vi "AutoAdjustCamera.vi"(8 "error in":errorcluster, 10 "Camera Settings":T1={"Brightness"=150, "Contrast"=0.2, "Threshold"=0.2}, 11 "Session In":T2) -> (0 "error out":errorcluster, 1 "Brightness":i64, 2 "Contrast":dbl, 3 "Session Out":T2, 4 "All Edges Found":bool, 5 "Threshold":sgl)   [LabVIEW 2017]
uses:
  <vilib>/userdefined/High Color/IMAQdx.ctl
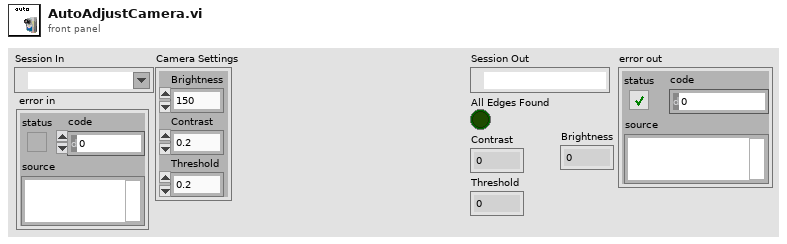
[diagram p1: front panel]
types:
  T1 = cluster{"Brightness":i64, "Contrast":dbl, "Threshold":sgl}
  T2 = typedef "IMAQdx.ctl" = refnum<k21>
  T3 = typedef "IMAQ Coordinate System" = cluster{"Reference System":cluster{"Origin":cluster{"X":sgl, "Y":sgl}, "Angle (deg)":sgl, "Axis Reference":u32}, "Measurement System":cluster{"Origin":cluster{"X":sgl, "Y":sgl}, "Angle (deg)":sgl, "Axis Reference":u32}}
  T4 = typedef "IMAQ Image.ctl" = refnum<image>
  T5 = cluster{"Point1 (Pixels)":cluster{"X":sgl, "Y":sgl}, "Point2 (Pixels)":cluster{"X":sgl, "Y":sgl}, "Point1 (Real-World)":cluster{"X":sgl, "Y":sgl}, "Point2 (Real-World)":cluster{"X":sgl, "Y":sgl}, "Angle (Pixel)":dbl, "Angle (Real-World)":dbl, "Score":dbl, "Straightness":dbl, "Average SNR (db)":dbl, "Calibration Valid":bool}[]
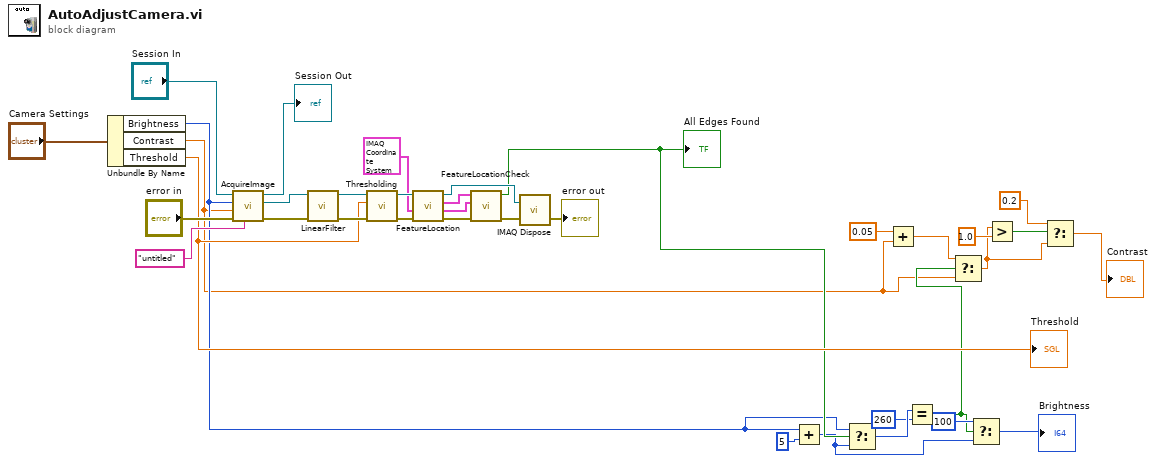
[diagram p0: block diagram]
diagram:
  n1 = Unbundle By Name("Camera Settings") -> ("Brightness"=w15:i64, "Contrast"=w8:dbl, "Threshold"=w20:sgl)
  "Threshold" <- w20
  n2 = call "AcquireImage.vi"("Image Name"="untitled", "error in"="error in", "Contrast"=w8, "Brightness"=w15, "Session In"="Session In") -> ("error out"=w32:errorcluster, "Image"=w31:T4, "Session Out"=→"Session Out":T2)  [unwired: 3 in]
  n3 = call "LinearFilter.vi"("error in (no error)"=w32, "Image Src"=w31) -> ("error out"=w26:errorcluster, "Image"=w25:T4)  [unwired: 8 in]
  n4 = call "Thresholding.vi"("error in (no error)"=w26, "Threshold Value"=w20, "Image Src"=w25) -> ("error out"=w28:errorcluster, "Image"=w27:T4)  [unwired: 7 in]
  n5 = call "FeatureLocation.vi"("error in (no error)"=w28, "Coordinate System"=T3 {"Reference System"={"Origin"={"X"=0.0, "Y"=0.0}, "Angle (deg)"=0.0, "Axis Reference"=0}, "Measurement System"={"Origin"={"X"=0.0, "Y"=0.0}, "Angle (deg)"=0.0, "Axis Reference"=0}}, "Image"=w27) -> ("error out"=w33:errorcluster, "Vertical Edges"=w30:T5, "Horizontal Edges"=w29:T5, "Image 2"=w35:T4)  [unwired: 3 in, 2 out]
  n6 = call "FeatureLocationCheck.vi"("error in (no error)"=w33, "Vertical Edges"=w30, "Horizontal Edges"=w29) -> ("error out"=w34:errorcluster, "All Edges Found"=w16:bool)  [unwired: 7 in]
  "All Edges Found" <- w16
  n7 = call "IMAQ Dispose"("Image"=w35, "error in (no error)"=w34) -> ("error out"=→"error out":errorcluster)  [unwired: 4 in]
  n8 = Add(x=w15, y=i64 5) -> (x+y=w11:i64)
  n9 = Select(t=w15, s=w16, f=w11) -> (s? t:f=w14:i64)
  n10 = Add(x=0.05, y=w8) -> (x+y=w6:dbl)
  n11 = Equal?(x=w14, y=i64 260) -> (x = y?=w9:bool)
  n12 = Select(t=w6, s=w9, f=w8) -> (s? t:f=w2:dbl)
  n13 = Select(t=i64 100, s=w9, f=w11) -> (s? t:f=→"Brightness":i64)
  n14 = Greater?(x=w2, y=1.0) -> (0:w4:bool)
  n15 = Select(t=0.2 ("f"), s=w4, f=w2) -> (s? t:f=→"Contrast":dbl)
